vi "多参校准读取.vi"(8 "Error in":errorcluster caption="Error in (no error)", 11 "站号":u16(ring)=10 items=["氨氮"=3, "水温"=9, "pH值"=10, "溶解氧"=11, "电导率"=12, "浊度"=13, "叶绿素a"=14, "藻密度"=15, "蓝绿藻"=16, "氧化还原电位"=17, "溶解氧%"=18, "盐度"=19]) -> (0 "error out":errorcluster, 2 "B":dbl caption="校准值B:", 3 "K":dbl caption="校准值K:")   [LabVIEW 2016, in "斯坦道原位多参数.lvlib"]
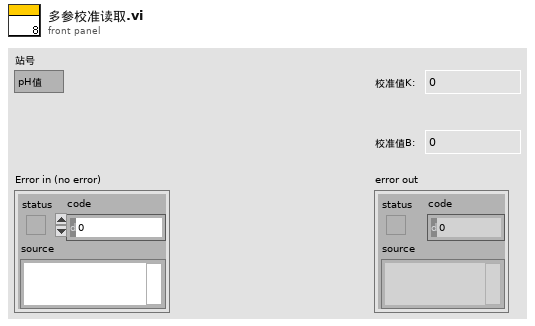
[diagram p1: front panel]
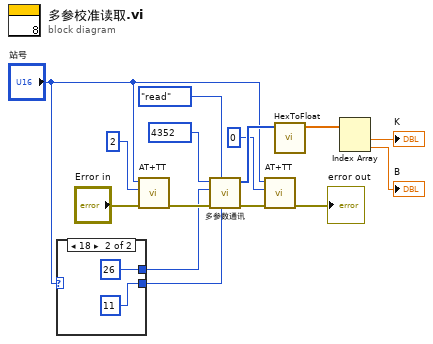
[diagram p0: block diagram]
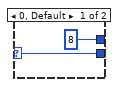
[diagram p2: hidden frame]
diagram:
  n1 = case shown="18" "站号" {
    selector: "站号" -> [w17 _]
    tunnel: [w17 u16 11 ("站号")] -> w7
    tunnel: [u16 8 ("quantity") u16 26 ("quantity")] -> w2
    frame 0, Default {
    }
    frame 18 {
    }
  }
  n2 = call "AT+TT.vi"("错误输入（无错误）"="Error in", "Count"=2, "站号"="站号") -> ("错误输出"=w8:errorcluster)  [unwired: 7 in, 1 out]
  n3 = call "多参数通讯.vi"("Slave ID"=w7, "STEP"=enum16{"open", "read", "write", "close"}."read", "Error in"=w8, "quantity"=w2, "starting address"=u16 4352) -> ("error out"=w6:errorcluster, "Registers"=w14:u16[])  [unwired: 4 in, 1 out]
  n4 = call "AT+TT.vi"("错误输入（无错误）"=w6, "Count"=0, "站号"="站号") -> ("错误输出"=→"error out":errorcluster)  [unwired: 7 in, 1 out]
  n5 = call "HexToFloat.vi"("数组"=w14) -> ("FLOAT"=w13:sgl[])  [unwired: 10 in]
  n6 = Index Array(array=w13) -> (element #1=→"K":sgl, element #2=→"B":sgl)  [unwired: 2 in]
